vi "Close.vi"(8 "error in (no error)":errorcluster, 11 "ICamera in":refnum<class "ICamera.lvclass">) -> (0 "error out":errorcluster, 3 "ICamera out":refnum<class "ICamera.lvclass">)   [LabVIEW 2023, in "HAL Interfaces.lvlib" / "ICamera.lvclass"]
uses:
  ICamera.lvclass
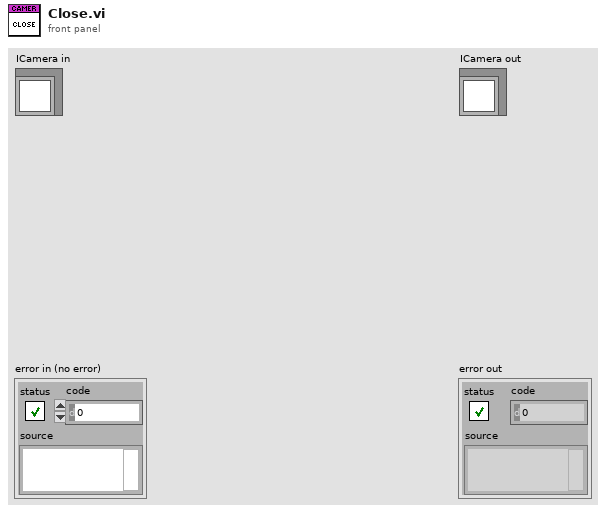
[diagram p1: front panel]
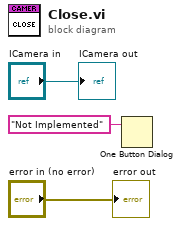
[diagram p0: block diagram]
diagram:
  n1 = One Button Dialog(message="Not Implemented") -> ()  [unwired: 1 in, 1 out]
  "error out" <- "error in (no error)"
  "ICamera out" <- "ICamera in"
